vi "Split into 3.vi"(0 "Cx":dbl[](array[numeric]), 5 "Cy":dbl[](array[numeric]), 7 "Ix":dbl[](array[numeric]), 9 "Iy":dbl[](array[numeric]), 11 "X":u8[](array[numeric])) -> (2 "C1x":dbl[](array[numeric]), 3 "C1y":dbl[](array[numeric]), 4 "C2x":dbl[](array[numeric]), 6 "C2y":dbl[](array[numeric]), 10 "C3x":dbl[](array[numeric]), 15 "C3y":dbl[](array[numeric]))   [LabVIEW 2021, in "d15.lvlib" / "Cave.lvclass"]
uses:
  Cave.lvclass
  Diamond/Diamond.lvclass
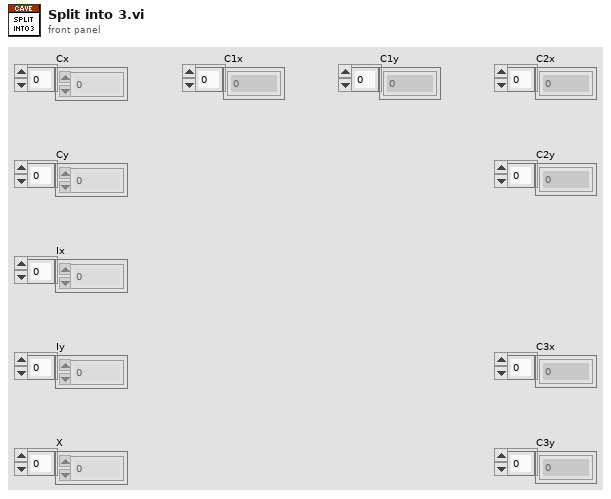
[diagram p1: front panel]
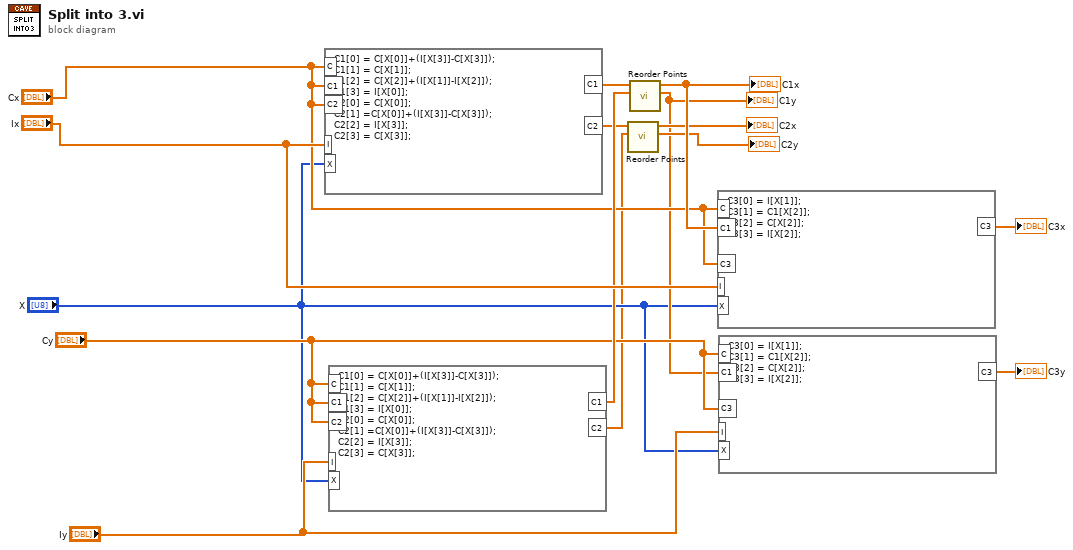
[diagram p0: block diagram]
diagram:
  n1 = formula code="C1[0] = C[X[0]]+(I[X[3]]-C[X[3]]);\nC1[1] = C[X[1]];\nC1[2] = C[X[2]]+(I[X[1]]-I[X[2]]);\nC1[3] = I[X[0]];\nC2[0] = C[X[0]];\nC2[1] =C[X[0]]+(I[X[3]]-C[X[3]]);\nC2[2] = I[X[3]];\nC2[3] = C[X[3]];"("C"="Cx", "I"="Ix", "X"="X", "C1"="Cx", "C2"="Cx") -> ("C1"=w14:dbl[], "C2"=w12:dbl[])
  n2 = formula code="C1[0] = C[X[0]]+(I[X[3]]-C[X[3]]);\nC1[1] = C[X[1]];\nC1[2] = C[X[2]]+(I[X[1]]-I[X[2]]);\nC1[3] = I[X[0]];\nC2[0] = C[X[0]];\nC2[1] =C[X[0]]+(I[X[3]]-C[X[3]]);\nC2[2] = I[X[3]];\nC2[3] = C[X[3]];"("C"="Cy", "I"="Iy", "X"="X", "C1"="Cy", "C2"="Cy") -> ("C1"=w13:dbl[], "C2"=w1:dbl[])
  n3 = call "Reorder Points.vi"("Y"=w1, "X"=w12) -> ("Y'"=→"C2y":dbl[], "X'"=→"C2x":dbl[])  [unwired: 8 in]
  n4 = call "Reorder Points.vi"("Y"=w13, "X"=w14) -> ("Y'"=w6:dbl[], "X'"=w11:dbl[])  [unwired: 8 in]
  "C1x" <- w11
  "C1y" <- w6
  n5 = formula code="C3[0] = I[X[1]];\nC3[1] = C1[X[2]];\nC3[2] = C[X[2]];\nC3[3] = I[X[2]];"("C"="Cx", "I"="Ix", "X"="X", "C1"=w11, "C3"="Cx") -> ("C3"=→"C3x":dbl[])
  n6 = formula code="C3[0] = I[X[1]];\nC3[1] = C1[X[2]];\nC3[2] = C[X[2]];\nC3[3] = I[X[2]];"("C"="Cy", "I"="Iy", "X"="X", "C1"=w6, "C3"="Cy") -> ("C3"=→"C3y":dbl[])
